vi "add subvi to vi.vi"(6 "position_y":i16, 8 "error in":errorcluster, 9 "position_x":i16, 10 "subvi_path":string, 11 "vi id":string) -> (0 "error out":errorcluster, 3 "ctl id":string)   [LabVIEW 2020]
doc: "Adds an object to the block diagram, structure sub-diagram or frontpanel of the referenced vi. Get a VI reference from new_vi or get a structure sub-diagram by get_stucture_diagram to add to this. If adding a control, consider the create_control tool and think about adding objects first and then creating structures around them using the enclose with selection.\nAdd a subVI or typedef by using the subvi_path, object name will be ignored. Leave subvi_path empty for all other objects."
uses:
  <vilib>/Utility/miscctls.llb/LVPointTypeDef.ctl
  G-AI Core/G-AI Core.lvlib
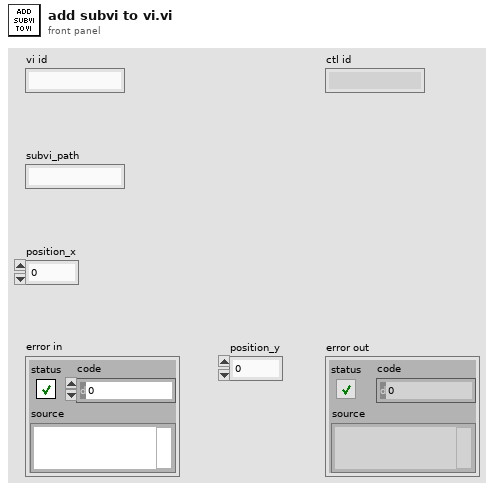
[diagram p1: front panel]
types:
  T1 = typedef "LVPointTypeDef.ctl" = cluster{"Horizontal":i16, "Vertical":i16}
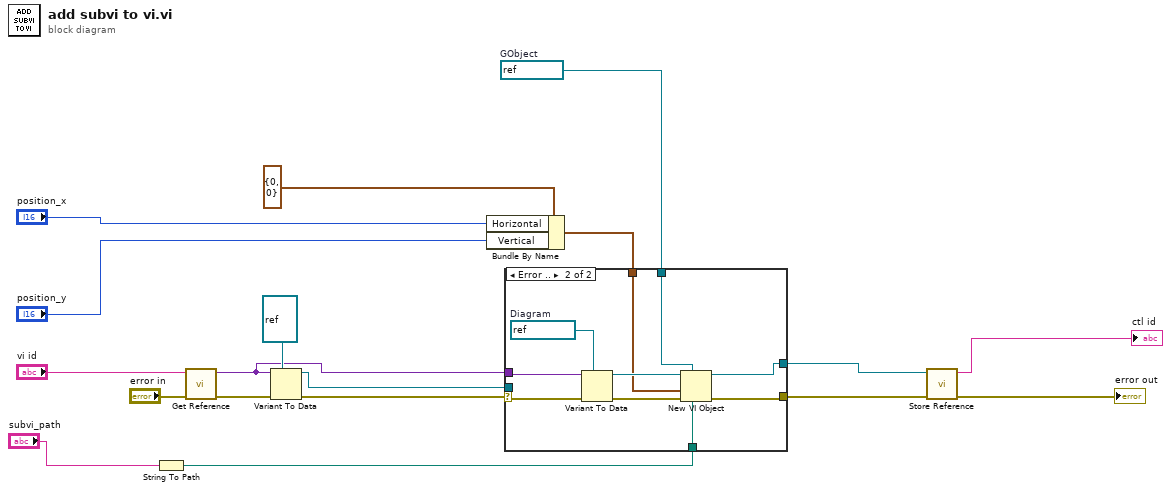
[diagram p0: block diagram]
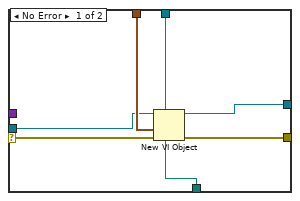
[diagram p2: hidden frame]
diagram:
  w7 = refnum<vi> refnum  # GObject
  n1 = String To Path(string="subvi_path") -> (path=w2:path)
  n2 = call "Get Reference.vi"("error in"="error in", "id"="vi id") -> ("error out"=w15:errorcluster, "reference"=w9:variant)  [unwired: 8 in]
  n3 = Variant To Data(error in=w15, type=refnum<vi> refnum ("vi reference"), Variant=w9) -> (data=w10:refnum<vi>, error out=w8:errorcluster)
  n4 = Bundle By Name(cluster=T1 {"Horizontal"=0, "Vertical"=0} ("location"), "Horizontal"="position_x", "Vertical"="position_y") -> (w6:T1)
  n5 = case shown="Error .." w8 {
    selector: w8 -> [w24 w35]
    tunnel: [w20 w31] -> w4
    tunnel: w10 -> [w22 _]
    tunnel: w9 -> [_ w33]
    tunnel: w7 -> [w25 w29]
    tunnel: w6 -> [w23 w28]
    tunnel: [w21 w27] -> w5
    tunnel: w2 -> [w19 w26]
    frame No Error {
      n6 = New VI Object(vi object class=w25, owner refnum=w22, position/next to=w23, 6:w19, 8:w24) -> (object refnum=w21:refnum<vi>, 0:w20:errorcluster)  [unwired: 3 in]
    }
    frame Error {
      w32 = refnum<vi> refnum  # Diagram
      n7 = Variant To Data(error in=w35, type=w32, Variant=w33) -> (data=w30:refnum<vi>, error out=w34:errorcluster)
      n8 = New VI Object(vi object class=w29, owner refnum=w30, position/next to=w28, 6:w26, 8:w34) -> (object refnum=w27:refnum<vi>, 0:w31:errorcluster)  [unwired: 3 in]
    }
  }
  n9 = call "Store Reference.vi"("error in"=w4, "Reference"=w5) -> ("error out"=→"error out":errorcluster, "id"=→"ctl id":string)  [unwired: 8 in]
